vi "Update FP.vi"(7 "defer fp updates (T)":bool=TRUE, 8 "error in (no error)":errorcluster, 9 "active wheel indexes in":i32[](array[numeric]), 10 "fp refs":T1, 11 "steering frame ref in":refnum<data-value>) -> (0 "error out":errorcluster, 3 "steering frame ref out":refnum<data-value>)   [LabVIEW 2017, in "NI_Robotics_Configure Steering Frame.lvlib" / "User Defined Frame Subpanel.lvlib"]
uses:
  <vilib>/robotics/Dialog/Configure Steering Frame/User Defined Frame Subpanel/User Defined Frame Subpanel.lvlib
  <vilib>/robotics/Dialog/Configure Steering Frame/User Defined Frame Subpanel/FP Refs.ctl
  <vilib>/robotics/Steering/Steering Frame/NI_Robotics_Steering Frame.lvclass
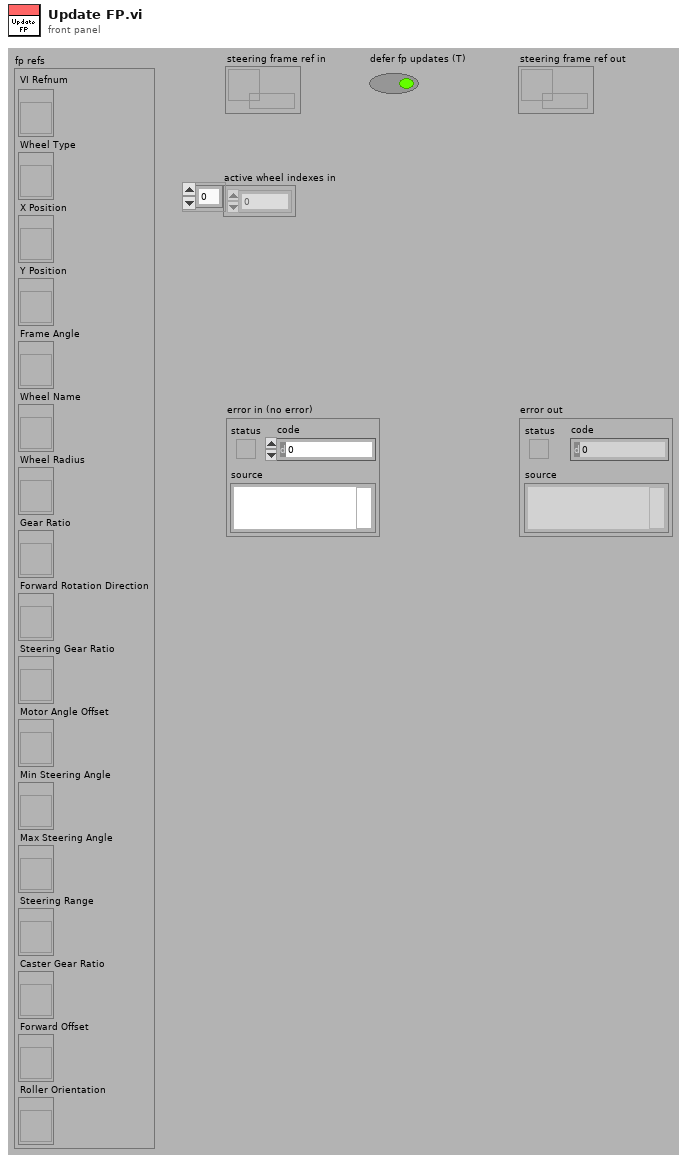
[diagram p1: front panel]
types:
  T1 = typedef "NI_Robotics_Configure Steering Frame.lvlib/User Defined Frame Subpanel.lvlib/FP Refs.ctl" = cluster{"VI Refnum":refnum<vi>, "Wheel Type":refnum<vi>, "X Position":refnum<vi>, "Y Position":refnum<vi>, "Frame Angle":refnum<vi>, "Wheel Name":refnum<vi>, "Wheel Radius":refnum<vi>, "Gear Ratio":refnum<vi>, "Forward Rotation Direction":refnum<vi>, "Steering Gear Ratio":refnum<vi>, "Motor Angle Offset":refnum<vi>, "Min Steering Angle":refnum<vi>, "Max Steering Angle":refnum<vi>, "Steering Range":refnum<vi>, "Caster Gear Ratio":refnum<vi>, "Forward Offset":refnum<vi>, "Roller Orientation":refnum<vi>}
  T2 = typedef "NI_Robotics_Configure Steering Frame.lvlib/User Defined Frame Subpanel.lvlib/Enabled Items.ctl" = cluster{"Wheel Type":bool, "X Position":bool, "Y Position":bool, "Frame Angle":bool, "Wheel Name":bool, "Wheel Radius":bool, "Gear Ratio":bool, "Forward Rotation Direction":bool, "Steering Gear Ratio":bool, "Motor Angle Offset":bool, "Min Steering Angle":bool, "Max Steering Angle":bool, "Steering Range":bool, "Caster Gear Ratio":bool, "Forward Offset":bool, "Roller Orientation":bool}
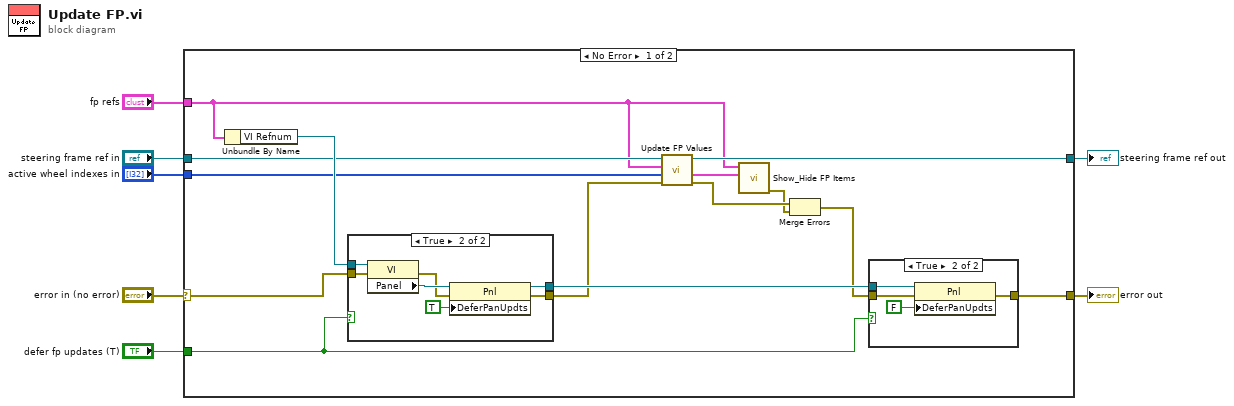
[diagram p0: block diagram]
diagram:
  n1 = case shown="No Error" "error in (no error)" {
    selector: "error in (no error)" -> [w20 w35]
    tunnel: [w18 w35] -> w7
    tunnel: "steering frame ref in" -> [w15 w36]
    tunnel: [w14 w36] -> w5
    tunnel: "fp refs" -> [w13 _]
    tunnel: "active wheel indexes in" -> [w16 _]
    tunnel: "defer fp updates (T)" -> [w17 _]
    frame No Error {
      n2 = Unbundle By Name(w13) -> ("VI Refnum"=w21:refnum<vi>)
      n3 = case shown="True" w17 {
        tunnel: [_ w32] -> w19
        tunnel: w21 -> [_ w31]
        tunnel: w20 -> [w27 w30]
        tunnel: [w27 w28] -> w12
        frame False {
        }
        frame True {
          n4 = property class="VI"(reference=w31, error in=w30) -> (error out=w29:errorcluster, "Panel"=w34:refnum<vi>)  [unwired: 1 out]
          n5 = property class="Pnl"(reference=w34, error in=w29, "DeferPanUpdts"=TRUE ("Defer Panel Updates")) -> (reference out=w32:refnum<vi>, error out=w28:errorcluster)
        }
      }
      n6 = call <vilib>:"Update FP Values.vi"("error in (no error)"=w12, "active wheel indexes in"=w16, "fp refs"=w13, "steering frame ref in"=w15) -> ("error out"=w10:errorcluster, "enabled items out"=w8:T2, "steering frame ref out"=w14:refnum<data-value>)  [unwired: 5 in]
      n7 = call <vilib>:"Show_Hide FP Items.vi"("active wheel types"=w8, "fp refs"=w13) -> ("error out"=w9:errorcluster)  [unwired: 9 in]
      n8 = Merge Errors(w10, w9) -> (w11:errorcluster)
      n9 = case shown="True" w17 {
        tunnel: w19 -> [_ w25]
        tunnel: w11 -> [w22 w24]
        tunnel: [w22 w23] -> w18
        frame False {
        }
        frame True {
          n10 = property class="Pnl"(reference=w25, error in=w24, "DeferPanUpdts"=FALSE ("Defer Panel Updates")) -> (error out=w23:errorcluster)  [unwired: 1 out]
        }
      }
    }
    frame Error {
    }
  }
  "error out" <- w7
  "steering frame ref out" <- w5
